vi "运维调试_五参数.vi"() -> ()   [LabVIEW 2016, in "斯坦道原位多参数.lvlib"]
uses:
  <vilib>/Utility/miscctls.llb/LVPointTypeDef.ctl
  <vilib>/Utility/config.llb/NI_LVConfig.lvlib
panel:
  in  "电导率单位":enum16{"mS/cm", "μS/cm"}(ring)
  in  "传感器类型":enum16{"STD自研", "纳清"}(ring)
  in  "校准":bool
  in  "获取传感器参数并保存触发":bool
  in  "传感器参数自动获取":bool=TRUE
  in  "标样测试组数":dbl=1.0 caption="标样测试组数:"
  in  "水样测试组数":dbl=1.0 caption="水样测试组数:"
  in  "转刷清洗时间":dbl=30.0 caption="转刷清洗时间:"
  in  "上电初始化时间":dbl=5.0 caption="上电初始化时间:"
  in  "水样稳定时间":dbl=5.0 caption="水样稳定时间:"
  out "串口号":string
  in  "水深写入":bool
  in  "水深读取":bool
  in  "水深校准":dbl caption="水深校准:"
  out "模块版本号":string
  in  "写入":bool
  in  "读取":bool
  in  "B":dbl caption="校准值B:"
  in  "K":dbl caption="校准值K:"
  in  "标样核查":bool
  in  "串口设置":bool
  in  "质控参数设置":bool
  in  "打开串口":bool
  in  "释放串口":bool
  out "多参数横条运行状态":T1(xcontrol)
  in  "数据区":i32(listbox)
  in  "停止测量(单探)":bool
  in  "启动测量(单探)":bool
  in  "控制命令区探头选择":u16(ring)=9 items=["氨氮"=3, "水温"=9, "pH值"=10, "溶解氧"=11, "电导率"=12, "浊度"=13, "叶绿素a"=14, "藻密度"=15, "蓝绿藻"=16, "氧化还原电位"=17, "溶解氧%"=18, "盐度"=19]
  in  "同步时间":bool
  in  "初始化(清洗)":bool
  in  "停止测量(全部)":bool
  in  "启动测量(全部)":bool
  in  "关键参数区读取":bool
  in  "关键参数区":i32(listbox)
  in  "传感器参数读取":bool
  in  "传感器区":i32(listbox)
  in  "返回":bool
  in  "设置":bool
  out "运行状态":string
  in  "停止":bool
  in  "水样测试":bool
  out "集成报警信息":string
  # "min"
  # "组"
  # "组"
  # "s"
  # "s"
  # "水深校准"
  # "控制命令区"
  # "探头校准"
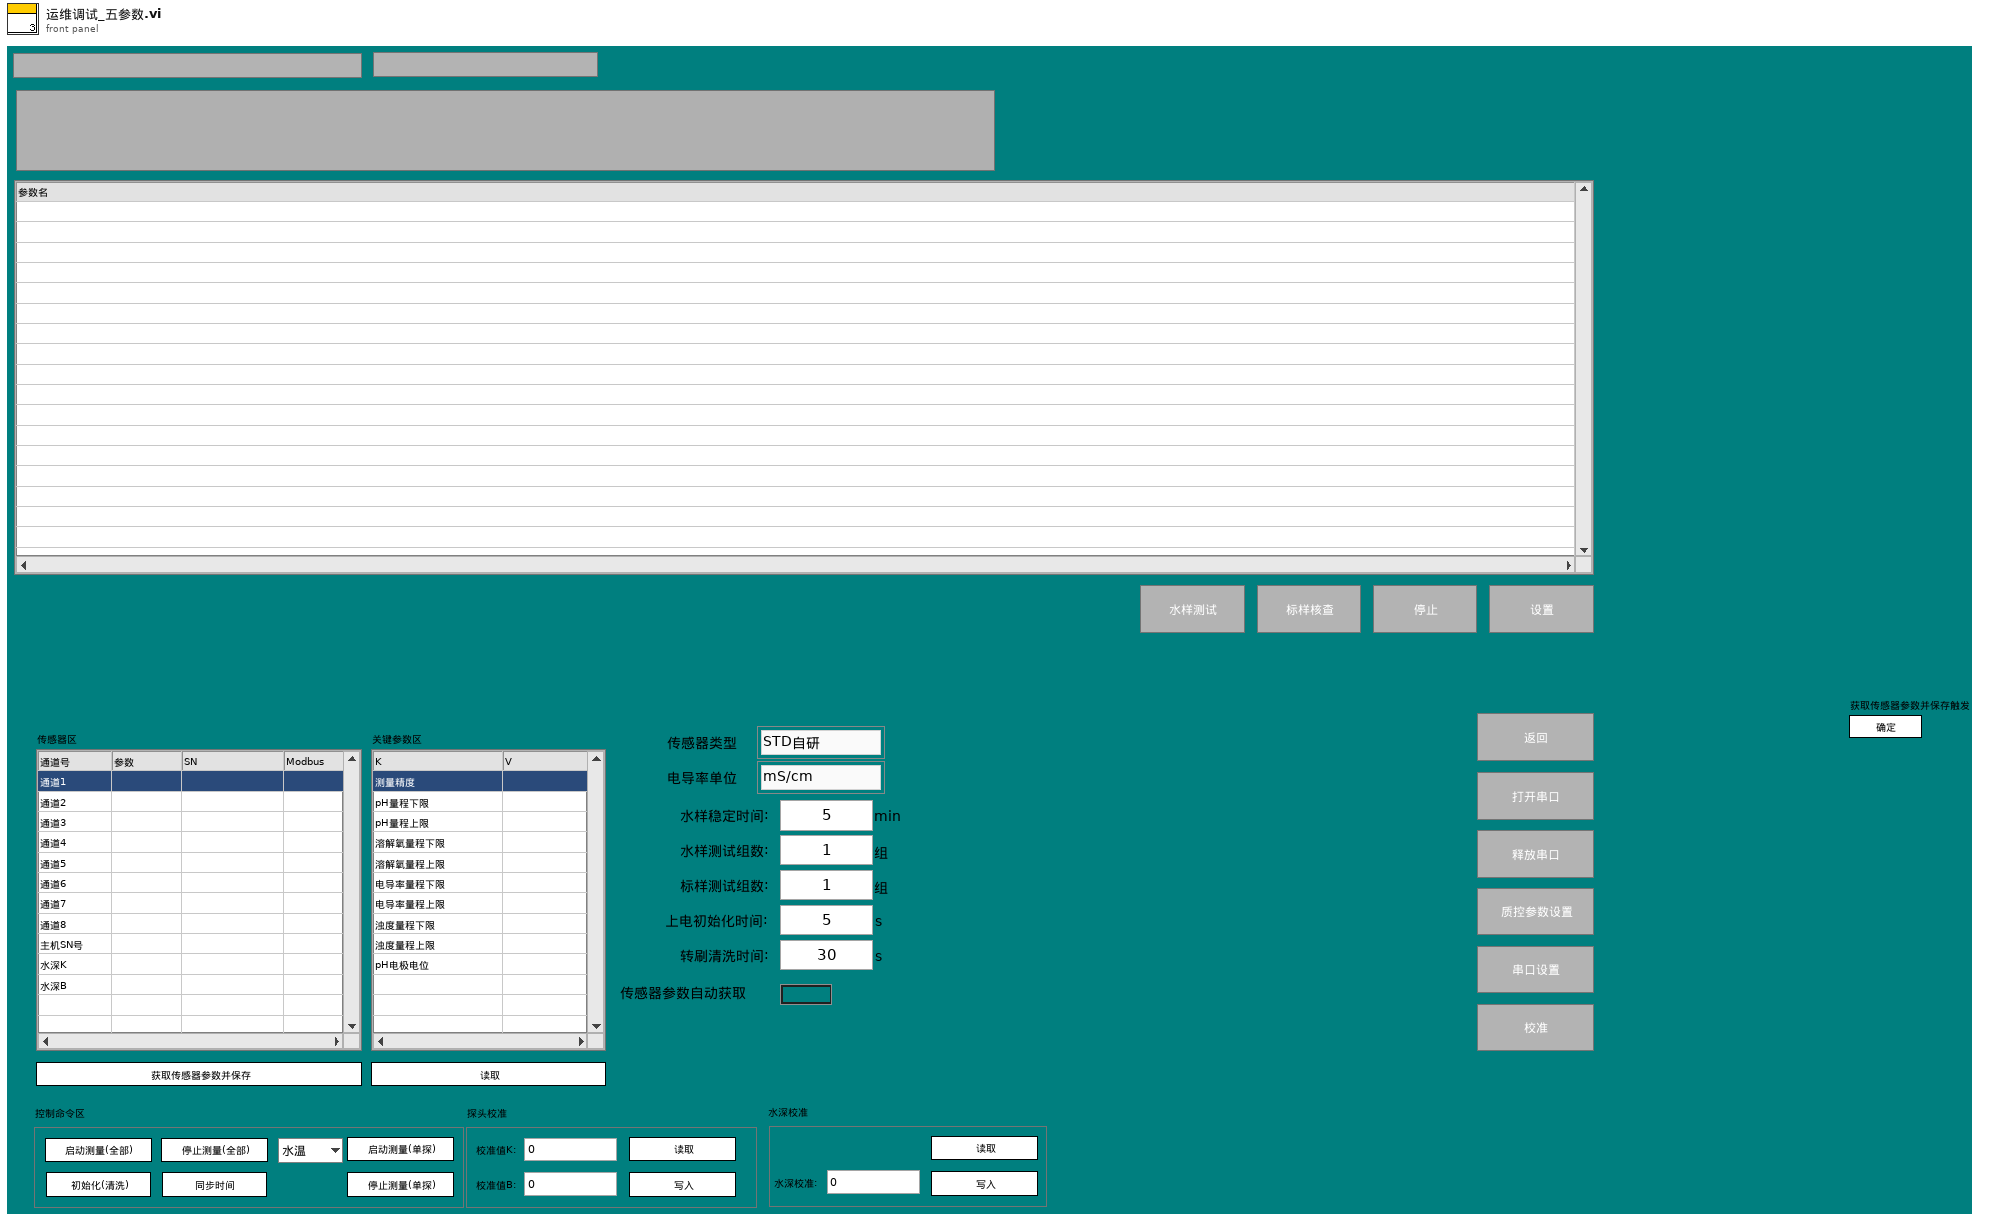
[diagram p1: front panel]
types:
  T1 = cluster{"系统时间":timestamp, "工作状态":u16, "测量模式":u16, "告警代码":enum16{"无告警", "缺试剂告警", "缺水样告警", "缺蒸馏水告警", "缺标液告警", "仪表漏液告警", "标定异常告警", "超量程告警", "加热异常", "低试剂预警", "超上限告警", "超下限告警", "仪表内部其他异常", "滴定异常告警", "电极异常告警", "量程切换告警", "参数设置告警", "PH电极电位异常", "电导率电极异常", "浊度光度异常", "溶解氧电极异常", "溶解氧光强异常", "温度异常告警", "PH异常告警", "溶解氧异常告警", "电导率异常告警", "浊度异常告警", "叶绿素异常告警", "藻密度异常告警", "蓝绿藻异常告警", "ORP异常告警", "氨氮异常告警", "清洁刷异常告警", "SD卡异常告警", "蓝牙异常告警", "Wifi异常告警", "流程异常告警"}, "故障代码":enum16{"无故障", "电机故障", "温度故障", "通讯故障", "滴定故障"}, "日志代码":u16, "软件版本":string}
  T2 = typedef "LVPointTypeDef.ctl" = cluster{"Horizontal":i16, "Vertical":i16}
  T3 = typedef "报警信息字段定义.ctl" = cluster{"时间":timestamp, "参数":string, "报警信息":string, "备注":string}
  T4 = enum16{"无告警", "缺试剂告警", "缺水样告警", "缺蒸馏水告警", "缺标液告警", "仪表漏液告警", "标定异常告警", "超量程告警", "加热异常", "低试剂预警", "超上限告警", "超下限告警", "仪表内部其他异常", "滴定异常告警", "电极异常告警", "量程切换告警", "参数设置告警", "PH电极电位异常", "电导率电极异常", "浊度光度异常", "溶解氧电极异常", "溶解氧光强异常", "温度异常告警", "PH异常告警", "溶解氧异常告警", "电导率异常告警", "浊度异常告警", "叶绿素异常告警", "藻密度异常告警", "蓝绿藻异常告警", "ORP异常告警", "氨氮异常告警", "清洁刷异常告警", "SD卡异常告警", "蓝牙异常告警", "Wifi异常告警", "流程异常告警"}
  T5 = cluster{"水温":dbl, "pH":dbl, "DO":dbl, "Cond":dbl, "Turb":dbl, "叶绿素":dbl, "藻密度":dbl, "蓝绿藻":dbl, "ORP":dbl, "NH3N":dbl}
  T6 = cluster{"因子编码":string, "单位":string, "标样参考值":sgl, "水样数据时间":timestamp, "水样实测值":sgl, "水样数据标识":string, "K":sgl, "B":sgl, "T":sgl, "H":sgl, "水深":sgl, "探头温度":sgl, "信号值":sgl}
  T7 = cluster{"Major":u16, "Minor":u16, "Fix":u16, "Build":u16}
  T8 = enum8{"Enabled", "Disabled", "Disabled and Grayed Out"}
  T9 = typedef "斯坦道原位多参数.lvlib/水样测试启动自定义输入参数.ctl" = cluster{"测量模式":string, "数据类型":string}
  T10 = typedef "斯坦道原位多参数.lvlib/标样核查启动自定义输入参数.ctl" = cluster{"测量模式":string, "数据类型":string, "输出参数":cluster{"水温":bool, "pH":bool, "DO":bool, "浊度":bool, "电导率":bool, "叶绿素a":bool, "蓝绿藻":bool, "藻密度":bool, "ORP":bool}}
  T11 = typedef "NI_LVConfig.lvlib/Config Data RefNum.ctl" = refnum<k1>
  T12 = cluster{"水温标准液标准浓度":dbl, "酸碱度标准液标准浓度":dbl, "溶解氧标准液标准浓度":dbl, "电导率标准液标准浓度":dbl, "浊度标准液标准浓度":dbl, "叶绿素a标准液标准浓度":dbl, "蓝绿藻标准液标准浓度":dbl, "ORP标准液标准浓度":dbl, "藻密度标准液标准浓度":dbl}
  T13 = cluster{"运行模式":enum16{"维护模式", "常规模式", "应急模式", "质控模式"}, "24H周期设置":bool[]}
  T14 = cluster{"水温":bool, "pH":bool, "DO":bool, "浊度":bool, "电导率":bool, "叶绿素a":bool, "蓝绿藻":bool, "藻密度":bool, "ORP":bool}
  T15 = enum32{"Bad", "Idle", "Run top level", "Running"}
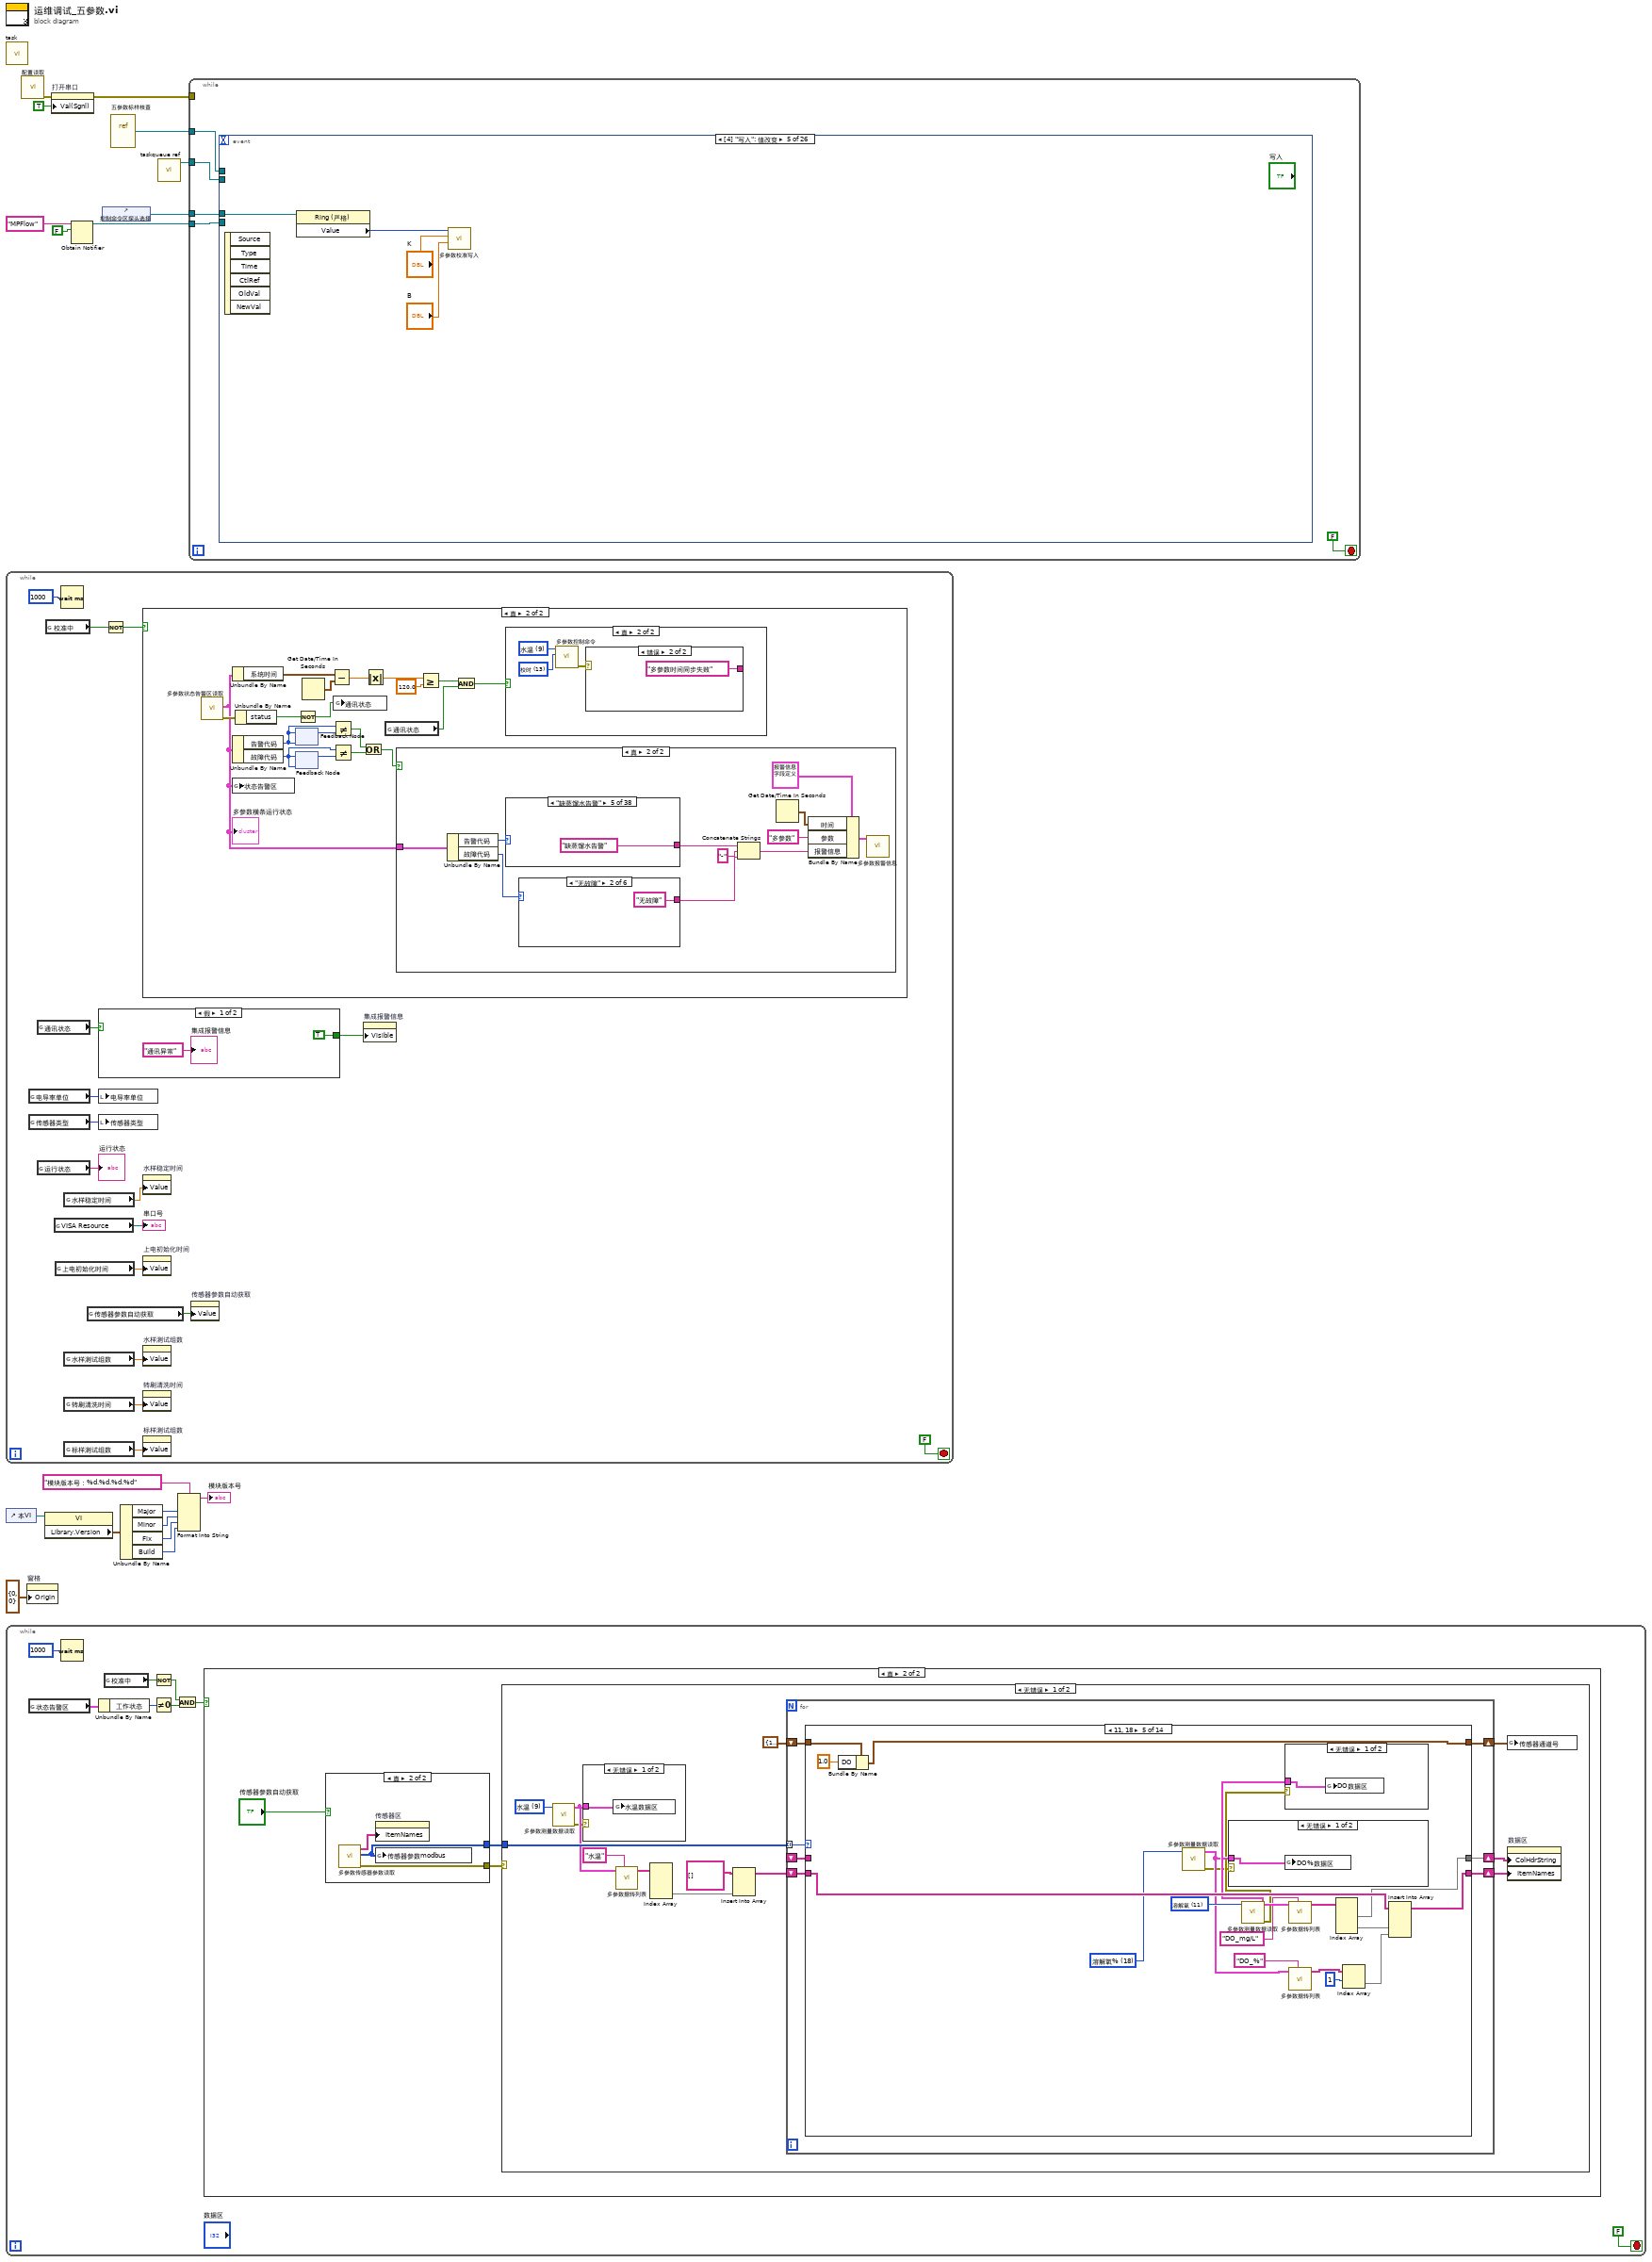
[diagram p0: block diagram]
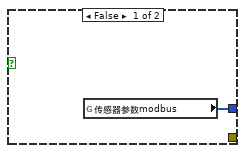
[diagram p3: hidden frame]
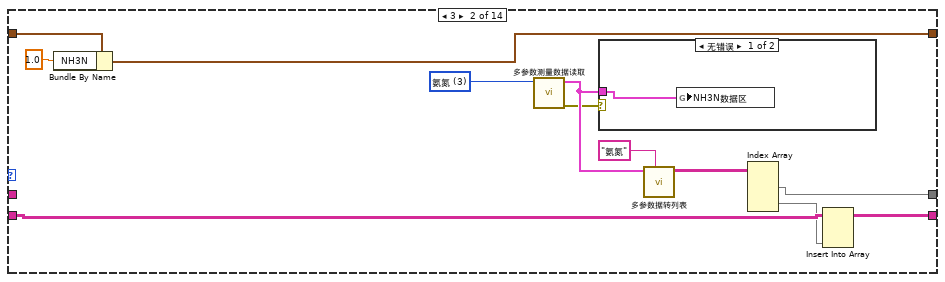
[diagram p6: hidden frame]
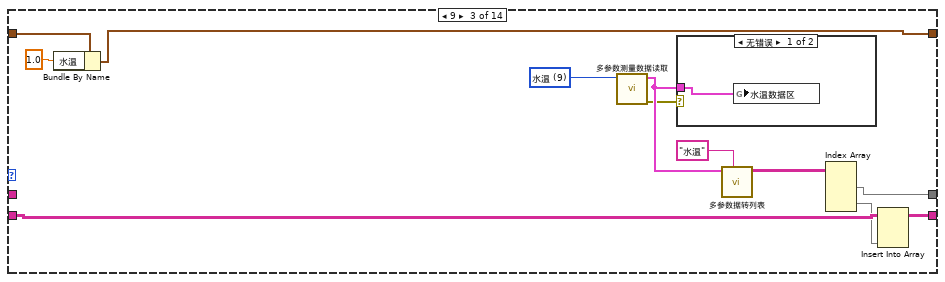
[diagram p8: hidden frame]
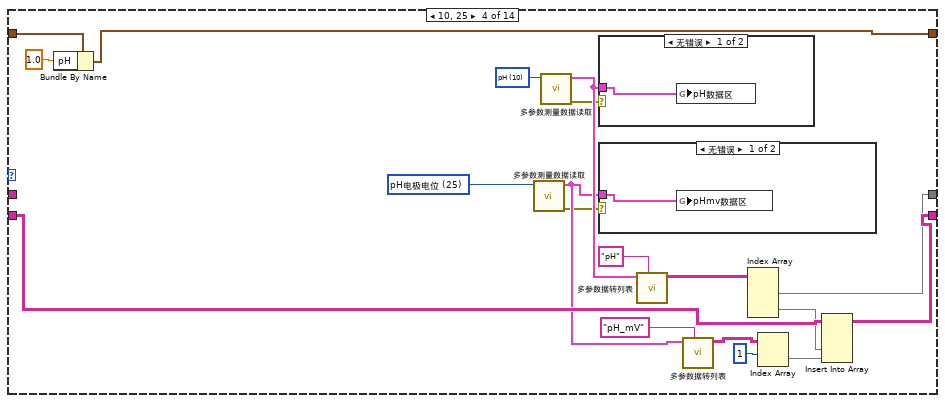
[diagram p10: hidden frame]
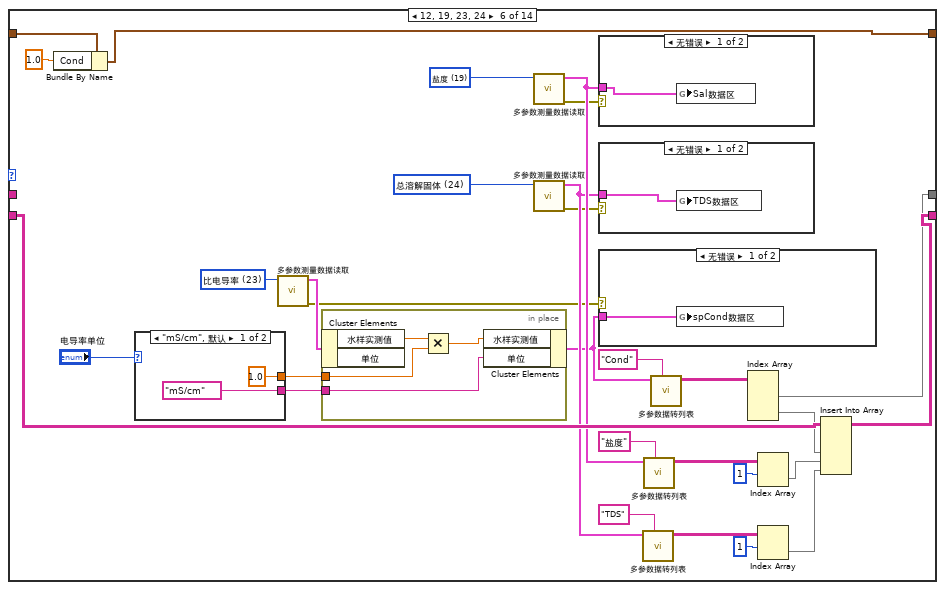
[diagram p15: hidden frame]
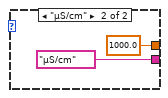
[diagram p16: hidden frame]
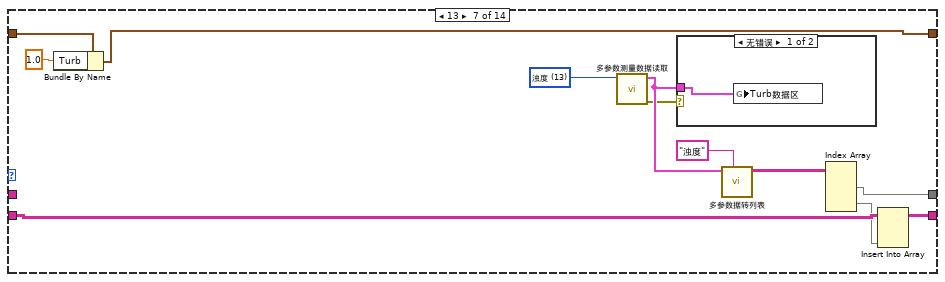
[diagram p20: hidden frame]
diagram:
  n1 = call "task.vi"() -> ()  [unwired: 12 in]
  n2 = while {
    stop <- FALSE stop-if-true
    n3 = global read "多参数断电保存全局变量.vi" "电导率单位"() -> (w21:enum16{"mS/cm", "μS/cm"})
    n4 = global read "多参数断电保存全局变量.vi" "传感器类型"() -> (w22:enum16{"STD自研", "纳清"})
    n5 = global read "多参数全局变量.vi" "通讯状态"() -> (w32:bool)
    n6 = global read "多参数全局变量.vi" "运行状态"() -> (→"运行状态":string)
    n7 = global read "多参数全局变量.vi" "校准中"() -> (w20:bool)
    n8 = global read "多参数断电保存全局变量.vi" "VISA Resource"() -> (→"串口号":refnum<visa-resource-name>)
    n9 = global read "多参数断电保存全局变量.vi" "上电初始化时间"() -> (w26:dbl)
    n10 = Wait (ms)(milliseconds to wait=u32 1000 ("等待时间（毫秒）")) -> ()  [unwired: 1 out]
    n11 = global read "多参数断电保存全局变量.vi" "水样稳定时间"() -> (w28:dbl)
    n12 = global read "多参数断电保存全局变量.vi" "水样测试组数"() -> (w27:dbl)
    n13 = global read "多参数断电保存全局变量.vi" "转刷清洗时间"() -> (w25:dbl)
    n14 = global read "多参数断电保存全局变量.vi" "标样测试组数"() -> (w24:dbl)
    n15 = global read "多参数断电保存全局变量.vi" "传感器参数自动获取"() -> (w23:bool)
    n16 = case shown="假" w32 {
      tunnel: [TRUE ("可见") _] -> w31
      frame False {
        "集成报警信息" <- "通讯异常" ("集成报警信息")
      }
      frame True {
      }
    }
    n17 = local write "电导率单位"(w21) -> ()
    n18 = local write "传感器类型"(w22) -> ()
    n19 = Not(x=w20) -> (.not. x?=w19:bool)
    n20 = case shown="真" w19 {
      frame False {
      }
      frame True {
        n21 = call "多参数状态告警区读取.vi"() -> ("error out"=w46:errorcluster, "状态告警块"=w43:T1)  [unwired: 9 in, 1 out]
        "多参数横条运行状态" <- w43
        n22 = Unbundle By Name(w43) -> ("系统时间"=w42:timestamp)
        n23 = Unbundle By Name(w43) -> ("告警代码"=w52:T4, "故障代码"=w50:enum16{"无故障", "电机故障", "温度故障", "通讯故障", "滴定故障"})
        n24 = global write "多参数全局变量.vi" "状态告警区"(w43) -> ()
        n25 = Unbundle By Name(w46) -> ("status"=w45:bool)
        n26 = feedback #1(w52) -> (w53:T4)
        n27 = feedback-in #1(w52) -> ()
        n28 = feedback #2(w50) -> (w51:enum16{"无故障", "电机故障", "温度故障", "通讯故障", "滴定故障"})
        n29 = feedback-in #2(w50) -> ()
        n30 = Not(x=w45) -> (.not. x?=w44:bool)
        n31 = Get Date/Time In Seconds() -> (seconds since 1Jan1904=w41:timestamp)
        n32 = Subtract(x=w42, y=w41) -> (x-y=w40:dbl)
        n33 = Not Equal?(x=w52, y=w53) -> (x != y?=w48:bool)
        n34 = Not Equal?(x=w50, y=w51) -> (x != y?=w49:bool)
        n35 = global write "多参数全局变量.vi" "通讯状态"(w44) -> ()
        n36 = Or(x=w48, y=w49) -> (x .or. y?=w47:bool)
        n37 = Absolute Value(x=w40) -> (abs(x)=w39:dbl)
        n38 = global read "多参数全局变量.vi" "通讯状态"() -> (w35:bool)
        n39 = case shown="真" w47 {
          tunnel: w43 -> [_ w69]
          frame False {
          }
          frame True {
            n40 = Unbundle By Name(w69) -> ("告警代码"=w68:T4, "故障代码"=w67:enum16{"无故障", "电机故障", "温度故障", "通讯故障", "滴定故障"})
            n41 = case shown="\"缺蒸馏水告警\"" w68 {
              selector: w68 -> [w80 _ _ _ _ _ _ _ _ _ _ _ _ _ _ _ _ _ _ _ _ _ _ _ _ _ _ _ _ _ _ _ _ _ _ _ _ _]
              tunnel: [w79 "无告警" "缺试剂告警" "缺水样告警" "缺蒸馏水告警" "缺标液告警" "仪表漏液告警" "标定异常告警" "超量程告警" "加热异常" "低试剂预警" "超上限告警" "超下限告警" "仪表内部其他异常" "滴定异常告警" "电极异常告警" "量程切换告警" "参数设置告警" "PH电极电位异常" "电导率电极异常" "浊度光度异常" "溶解氧电极异常" "溶解氧光强异常" "温度异常告警" "PH异常告警" "溶解氧异常告警" "电导率异常告警" "浊度异常告警" "叶绿素异常告警" "藻密度异常告警" "蓝绿藻异常告警" "ORP异常告警" "氨氮异常告警" "清洁刷异常告警" "SD卡异常告警" "蓝牙异常告警" "WiFi异常告警" "流程异常告警"] -> w66
              frame Default {
                n42 = Format Into String(format string="%d" ("格式字符串"), initial string="未知" ("工作状态"), w80) -> (resulting string=w79:string)  [unwired: 1 in, 1 out]
              }
              frame "无告警" {
              }
              frame "缺试剂告警" {
              }
              frame "缺水样告警" {
              }
              frame "缺蒸馏水告警" {
              }
              frame "缺标液告警" {
              }
              frame "仪表漏液告警" {
              }
              frame "标定异常告警" {
              }
              frame "超量程告警" {
              }
              frame "加热异常" {
              }
              frame "低试剂预警" {
              }
              frame "超上限告警" {
              }
              frame "超下限告警" {
              }
              frame "仪表内部其他异常" {
              }
              frame "滴定异常告警" {
              }
              frame "电极异常告警" {
              }
              frame "量程切换告警" {
              }
              frame "参数设置告警" {
              }
              frame "PH电极电位异常" {
              }
              frame "电导率电极异常" {
              }
              frame "浊度光度异常" {
              }
              frame "溶解氧电极异常" {
              }
              frame "溶解氧光强异常" {
              }
              frame "温度异常告警" {
              }
              frame "PH异常告警" {
              }
              frame "溶解氧异常告警" {
              }
              frame "电导率异常告警" {
              }
              frame "浊度异常告警" {
              }
              frame "叶绿素异常告警" {
              }
              frame "藻密度异常告警" {
              }
              frame "蓝绿藻异常告警" {
              }
              frame "ORP异常告警" {
              }
              frame "氨氮异常告警" {
              }
              frame "清洁刷异常告警" {
              }
              frame "SD卡异常告警" {
              }
              frame "蓝牙异常告警" {
              }
              frame "Wifi异常告警" {
              }
              frame "流程异常告警" {
              }
            }
            n43 = case shown="\"无故障\"" w67 {
              selector: w67 -> [w71 _ _ _ _ _]
              tunnel: [w70 "无故障" "电机故障" "温度故障" "通讯故障" "滴定故障"] -> w65
              frame Default {
                n44 = Format Into String(format string="%d" ("格式字符串"), initial string="未知" ("工作状态"), w71) -> (resulting string=w70:string)  [unwired: 1 in, 1 out]
              }
              frame "无故障" {
              }
              frame "电机故障" {
              }
              frame "温度故障" {
              }
              frame "通讯故障" {
              }
              frame "滴定故障" {
              }
            }
            n45 = Concatenate Strings(w66, "-" ("字符串"), w65) -> (w63:string)
            n46 = Get Date/Time In Seconds() -> (seconds since 1Jan1904=w62:timestamp)
            n47 = Bundle By Name(cluster=T3 {"时间"=timestamp(0 s since 1904-01-01), "参数"="", "报警信息"="", "备注"=""} ("data"), "时间"=w62, "参数"="多参数" ("设备"), "报警信息"=w63) -> (w59:T3)
            n48 = call "多参数报警信息.vi"("data"=w59) -> ()  [unwired: 10 in, 1 out]
          }
        }
        n49 = Greater Or Equal?(x=w39, y=120.0) -> (x >= y?=w38:bool)
        n50 = And(x=w38, y=w35) -> (x .and. y?=w36:bool)
        n51 = case shown="真" w36 {
          frame False {
          }
          frame True {
            w54 = u16 13 items=["启动测量（全部）"=1, "初始化（清洗）"=10, "停止测量（全部）"=11, "校时"=13, "启动测量（单个传感器）"=19, "停止测量（单个传感器）"=20] ("控制命令")
            w55 = u16 9 items=["氨氮"=3, "水温"=9, "pH值"=10, "溶解氧"=11, "电导率"=12, "浊度"=13, "叶绿素a"=14, "藻密度"=15, "蓝绿藻"=16, "氧化还原电位"=17, "溶解氧%"=18, "盐度"=19] ("站号")
            n52 = call "多参数控制命令.vi"("控制命令"=w54, "站号"=w55) -> ("error out"=w56:errorcluster)  [unwired: 9 in]
            n53 = case shown="错误" w56 {
              tunnel: ["多参数时间同步成功" ("消息") "多参数时间同步失败" ("消息")] -> _
              frame No Error {
              }
              frame Error {
              }
            }
          }
        }
      }
    }
    n54 = property on="水样稳定时间" class="DigNum (严格)"("Value"=w28) -> ()  [unwired: 2 in, 2 out]
    n55 = property on="上电初始化时间" class="DigNum (严格)"("Value"=w26) -> ()  [unwired: 2 in, 2 out]
    n56 = property on="水样测试组数" class="DigNum (严格)"("Value"=w27) -> ()  [unwired: 2 in, 2 out]
    n57 = property on="转刷清洗时间" class="DigNum (严格)"("Value"=w25) -> ()  [unwired: 2 in, 2 out]
    n58 = property on="标样测试组数" class="DigNum (严格)"("Value"=w24) -> ()  [unwired: 2 in, 2 out]
    n59 = property on="传感器参数自动获取" class="Bool (严格)"("Value"=w23) -> ()  [unwired: 2 in, 2 out]
    n60 = property on="集成报警信息" class="Str"("Visible"=w31) -> ()  [unwired: 2 in, 2 out]
  }
  n61 = control-ref of="本VI"() -> (w10:refnum<vi>)
  n62 = while {
    stop <- FALSE stop-if-true
    n63 = global read "多参数全局变量.vi" "状态告警区"() -> (w127:T1)
    n64 = Wait (ms)(milliseconds to wait=u32 1000 ("等待时间（毫秒）")) -> ()  [unwired: 1 out]
    n65 = Unbundle By Name(w127) -> ("工作状态"=w126:u16)
    n66 = global read "多参数全局变量.vi" "校准中"() -> (w124:bool)
    n67 = Not(x=w124) -> (.not. x?=w122:bool)
    n68 = Not Equal To 0?(x=w126) -> (x != 0?=w125:bool)
    n69 = And(x=w122, y=w125) -> (x .and. y?=w123:bool)
    n70 = case shown="真" w123 {
      frame False {
      }
      frame True {
        n71 = case shown="真" "传感器参数自动获取" {
          tunnel: [_ w136] -> w132
          tunnel: [w133 w134] -> w131
          frame False {
            n72 = global read "多参数断电保存全局变量.vi" "传感器参数modbus"() -> (w133:u16[])
          }
          frame True {
            n73 = call "多参数传感器参数读取.vi"() -> ("error out"=w136:errorcluster, "modbus"=w134:u16[], "添加的数组"=w135:string[][])  [unwired: 9 in]
            n74 = property on="传感器区" class="MCListbox (严格)"("ItemNames"=w135) -> ()  [unwired: 2 in, 2 out]
            n75 = global write "多参数断电保存全局变量.vi" "传感器参数modbus"(w134) -> ()
          }
        }
        n76 = case shown="无错误" w132 {
          tunnel: w131 -> [w149 _]
          frame No Error {
            w146 = u16 9 items=["氨氮"=3, "水温"=9, "pH"=10, "溶解氧"=11, "电导率"=12, "浊度"=13, "叶绿素a"=14, "藻密度"=15, "蓝绿藻"=16, "氧化还原电位"=17, "溶解氧%"=18, "盐度"=19, "水中油"=20, "高锰酸盐指数"=21, "化学需氧量"=22, "比电导率"=23, "总溶解固体"=24, "pH电极电位"=25] ("下拉列表")
            n77 = call "多参数测量数据读取.vi"("探头选择"=w146) -> ("error out"=w137:errorcluster, "测量数据块"=w141:T6)  [unwired: 8 in, 1 out]
            n78 = case shown="无错误" w137 {
              tunnel: w141 -> [w150 _]
              frame No Error {
                n79 = global write "多参数全局变量.vi" "水温数据区"(w150) -> ()
              }
              frame Error {
              }
            }
            n80 = call "多参数据转列表.vi"("参数名"="水温", "测量数据块"=w141) -> ("添加的数组"=w139:string[][])  [unwired: 9 in]
            n81 = Index Array(array=w139) -> (element #2=w138:string[])  [unwired: 4 in, 1 out]
            n82 = Insert Into Array(array=string[][] [] ("子数组"), new element=w138) -> (w144:string[][])  [unwired: 2 in]
            n83 = for {
              tunnel: w149 -> [w157] mode=indexing
              shift-right: [w155] -> w147
              shift-left: w144 -> [w156]
              shift-right: [w154] -> w148
              shift-left: _ -> [w153]
              shift-right: [w152] -> w142
              shift-left: T5 {"水温"=1.0, "pH"=0.0, "DO"=0.0, "Cond"=0.0, "Turb"=0.0, "叶绿素"=0.0, "藻密度"=0.0, "蓝绿藻"=0.0, "ORP"=0.0, "NH3N"=0.0} ("传感器通道号") -> [w151]
              n84 = case shown="11, 18" w157 {
                tunnel: w156 -> [w160 w171 w184 w204 w225 w257 w280 w293 w306 w319 w332 w342 w351 w360]
                tunnel: [w160 w170 w183 w203 w224 w256 w279 w292 w305 w318 w331 w341 w350 w359] -> w155
                tunnel: [w159 w163 w176 w196 w217 w248 w273 w285 w300 w312 w325 w336 w345 w354] -> w154
                tunnel: w153 -> [w159 _ _ _ _ _ _ _ _ _ _ _ _ _]
                tunnel: [w158 w167 w180 w199 w221 w251 w276 w289 w302 w315 w328 w340 w349 w358] -> w152
                tunnel: w151 -> [w158 w169 w182 w201 w223 w252 w277 w290 w303 w316 w329 w340 w349 w358]
                frame 0, Default {
                }
                frame 3 {
                  w172 = u16 3 items=["氨氮"=3, "水温"=9, "pH"=10, "溶解氧"=11, "电导率"=12, "浊度"=13, "叶绿素a"=14, "藻密度"=15, "蓝绿藻"=16, "氧化还原电位"=17, "溶解氧%"=18, "盐度"=19, "水中油"=20, "高锰酸盐指数"=21, "化学需氧量"=22, "比电导率"=23, "总溶解固体"=24, "pH电极电位"=25] ("下拉列表")
                  n85 = Bundle By Name(cluster=w169, "NH3N"=1.0) -> (w167:T5)
                  n86 = call "多参数测量数据读取.vi"("探头选择"=w172) -> ("error out"=w161:errorcluster, "测量数据块"=w166:T6)  [unwired: 8 in, 1 out]
                  n87 = case shown="无错误" w161 {
                    tunnel: w166 -> [w173 _]
                    frame No Error {
                      n88 = global write "多参数全局变量.vi" "NH3N数据区"(w173) -> ()
                    }
                    frame Error {
                    }
                  }
                  n89 = call "多参数据转列表.vi"("参数名"="氨氮", "测量数据块"=w166) -> ("添加的数组"=w165:string[][])  [unwired: 9 in]
                  n90 = Index Array(array=w165) -> (element #1=w163:string[], element #2=w162:string[])  [unwired: 4 in]
                  n91 = Insert Into Array(array=w171, new element=w162) -> (w170:string[][])  [unwired: 2 in]
                }
                frame 9 {
                  w185 = u16 9 items=["氨氮"=3, "水温"=9, "pH"=10, "溶解氧"=11, "电导率"=12, "浊度"=13, "叶绿素a"=14, "藻密度"=15, "蓝绿藻"=16, "氧化还原电位"=17, "溶解氧%"=18, "盐度"=19, "水中油"=20, "高锰酸盐指数"=21, "化学需氧量"=22, "比电导率"=23, "总溶解固体"=24, "pH电极电位"=25] ("下拉列表")
                  n92 = Bundle By Name(cluster=w182, "水温"=1.0) -> (w180:T5)
                  n93 = call "多参数测量数据读取.vi"("探头选择"=w185) -> ("error out"=w174:errorcluster, "测量数据块"=w179:T6)  [unwired: 8 in, 1 out]
                  n94 = case shown="无错误" w174 {
                    tunnel: w179 -> [w186 _]
                    frame No Error {
                      n95 = global write "多参数全局变量.vi" "水温数据区"(w186) -> ()
                    }
                    frame Error {
                    }
                  }
                  n96 = call "多参数据转列表.vi"("参数名"="水温", "测量数据块"=w179) -> ("添加的数组"=w178:string[][])  [unwired: 9 in]
                  n97 = Index Array(array=w178) -> (element #1=w176:string[], element #2=w175:string[])  [unwired: 4 in]
                  n98 = Insert Into Array(array=w184, new element=w175) -> (w183:string[][])  [unwired: 2 in]
                }
                frame 10, 25 {
                  w202 = u16 25 items=["氨氮"=3, "水温"=9, "pH"=10, "溶解氧"=11, "电导率"=12, "浊度"=13, "叶绿素a"=14, "藻密度"=15, "蓝绿藻"=16, "氧化还原电位"=17, "溶解氧%"=18, "盐度"=19, "水中油"=20, "高锰酸盐指数"=21, "化学需氧量"=22, "比电导率"=23, "总溶解固体"=24, "pH电极电位"=25] ("下拉列表")
                  w205 = u16 10 items=["氨氮"=3, "水温"=9, "pH"=10, "溶解氧"=11, "电导率"=12, "浊度"=13, "叶绿素a"=14, "藻密度"=15, "蓝绿藻"=16, "氧化还原电位"=17, "溶解氧%"=18, "盐度"=19, "水中油"=20, "高锰酸盐指数"=21, "化学需氧量"=22, "比电导率"=23, "总溶解固体"=24, "pH电极电位"=25] ("下拉列表")
                  n99 = Bundle By Name(cluster=w201, "pH"=1.0) -> (w199:T5)
                  n100 = call "多参数测量数据读取.vi"("探头选择"=w202) -> ("error out"=w187:errorcluster, "测量数据块"=w192:T6)  [unwired: 8 in, 1 out]
                  n101 = call "多参数测量数据读取.vi"("探头选择"=w205) -> ("error out"=w188:errorcluster, "测量数据块"=w198:T6)  [unwired: 8 in, 1 out]
                  n102 = case shown="无错误" w188 {
                    tunnel: w198 -> [w207 _]
                    frame No Error {
                      n103 = global write "多参数全局变量.vi" "pH数据区"(w207) -> ()
                    }
                    frame Error {
                    }
                  }
                  n104 = case shown="无错误" w187 {
                    tunnel: w192 -> [w206 _]
                    frame No Error {
                      n105 = global write "多参数全局变量.vi" "pHmv数据区"(w206) -> ()
                    }
                    frame Error {
                    }
                  }
                  n106 = call "多参数据转列表.vi"("参数名"="pH", "测量数据块"=w198) -> ("添加的数组"=w197:string[][])  [unwired: 9 in]
                  n107 = call "多参数据转列表.vi"("参数名"="pH_mV", "测量数据块"=w192) -> ("添加的数组"=w191:string[][])  [unwired: 9 in]
                  n108 = Index Array(array=w197) -> (element #1=w196:string[], element #2=w195:string[])  [unwired: 4 in]
                  n109 = Index Array(array=w191, index (row)=1 ("禁用的索引 (列)")) -> (element=w194:string[])  [unwired: 1 in]
                  n110 = Insert Into Array(array=w204, new element #1=w195, new element #2=w194) -> (w203:string[][])  [unwired: 2 in]
                }
                frame 11, 18 {
                  w215 = u16 18 items=["氨氮"=3, "水温"=9, "pH"=10, "溶解氧"=11, "电导率"=12, "浊度"=13, "叶绿素a"=14, "藻密度"=15, "蓝绿藻"=16, "氧化还原电位"=17, "溶解氧%"=18, "盐度"=19, "水中油"=20, "高锰酸盐指数"=21, "化学需氧量"=22, "比电导率"=23, "总溶解固体"=24, "pH电极电位"=25] ("下拉列表")
                  w226 = u16 11 items=["氨氮"=3, "水温"=9, "pH"=10, "溶解氧"=11, "电导率"=12, "浊度"=13, "叶绿素a"=14, "藻密度"=15, "蓝绿藻"=16, "氧化还原电位"=17, "溶解氧%"=18, "盐度"=19, "水中油"=20, "高锰酸盐指数"=21, "化学需氧量"=22, "比电导率"=23, "总溶解固体"=24, "pH电极电位"=25] ("下拉列表")
                  n111 = Bundle By Name(cluster=w223, "DO"=1.0) -> (w221:T5)
                  n112 = call "多参数测量数据读取.vi"("探头选择"=w215) -> ("error out"=w208:errorcluster, "测量数据块"=w214:T6)  [unwired: 8 in, 1 out]
                  n113 = case shown="无错误" w208 {
                    tunnel: w214 -> [w227 _]
                    frame No Error {
                      n114 = global write "多参数全局变量.vi" "DO%数据区"(w227) -> ()
                    }
                    frame Error {
                    }
                  }
                  n115 = call "多参数测量数据读取.vi"("探头选择"=w226) -> ("error out"=w209:errorcluster, "测量数据块"=w220:T6)  [unwired: 8 in, 1 out]
                  n116 = case shown="无错误" w209 {
                    tunnel: w220 -> [w228 _]
                    frame No Error {
                      n117 = global write "多参数全局变量.vi" "DO数据区"(w228) -> ()
                    }
                    frame Error {
                    }
                  }
                  n118 = call "多参数据转列表.vi"("参数名"="DO_mg/L", "测量数据块"=w220) -> ("添加的数组"=w218:string[][])  [unwired: 9 in]
                  n119 = call "多参数据转列表.vi"("参数名"="DO_%", "测量数据块"=w214) -> ("添加的数组"=w212:string[][])  [unwired: 9 in]
                  n120 = Index Array(array=w218) -> (element #1=w217:string[], element #2=w216:string[])  [unwired: 4 in]
                  n121 = Index Array(array=w212, index (row)=1 ("禁用的索引 (列)")) -> (element=w211:string[])  [unwired: 1 in]
                  n122 = Insert Into Array(array=w225, new element #1=w216, new element #2=w211) -> (w224:string[][])  [unwired: 2 in]
                }
                frame 12, 19, 23, 24 {
                  w254 = u16 24 items=["氨氮"=3, "水温"=9, "pH"=10, "溶解氧"=11, "电导率"=12, "浊度"=13, "叶绿素a"=14, "藻密度"=15, "蓝绿藻"=16, "氧化还原电位"=17, "溶解氧%"=18, "盐度"=19, "水中油"=20, "高锰酸盐指数"=21, "化学需氧量"=22, "比电导率"=23, "总溶解固体"=24, "pH电极电位"=25] ("下拉列表")
                  w255 = u16 19 items=["氨氮"=3, "水温"=9, "pH"=10, "溶解氧"=11, "电导率"=12, "浊度"=13, "叶绿素a"=14, "藻密度"=15, "蓝绿藻"=16, "氧化还原电位"=17, "溶解氧%"=18, "盐度"=19, "水中油"=20, "高锰酸盐指数"=21, "化学需氧量"=22, "比电导率"=23, "总溶解固体"=24, "pH电极电位"=25] ("下拉列表")
                  w258 = u16 23 items=["氨氮"=3, "水温"=9, "pH"=10, "溶解氧"=11, "电导率"=12, "浊度"=13, "叶绿素a"=14, "藻密度"=15, "蓝绿藻"=16, "氧化还原电位"=17, "溶解氧%"=18, "盐度"=19, "水中油"=20, "高锰酸盐指数"=21, "化学需氧量"=22, "比电导率"=23, "总溶解固体"=24, "pH电极电位"=25] ("下拉列表")
                  n123 = Bundle By Name(cluster=w252, "Cond"=1.0 ("DO")) -> (w251:T5)
                  n124 = case shown="\"mS/cm\", 默认" "电导率单位" {
                    tunnel: ["mS/cm" ("单位") "μS/cm" ("单位")] -> w230
                    tunnel: [sgl 1.0 ("y") sgl 1000.0 ("y")] -> w229
                    frame "mS/cm", Default {
                    }
                    frame "μS/cm" {
                    }
                  }
                  n125 = call "多参数测量数据读取.vi"("探头选择"=w258) -> ("error out"=w234:errorcluster, "测量数据块"=w240:T6)  [unwired: 8 in, 1 out]
                  n126 = in-place {
                    in-place-border: w230 -> [w267]
                    in-place-border: w229 -> [w266]
                    n127 = in-place-cluster #3(w240) -> ("水样实测值"=w269:sgl)  [unwired: 1 out]
                    n128 = Multiply(x=w269, y=w266) -> (x*y=w268:sgl)
                    n129 = in-place-cluster #3("水样实测值"=w268, "单位"=w267) -> (w239:T6)
                  }
                  n130 = call "多参数测量数据读取.vi"("探头选择"=w255) -> ("error out"=w233:errorcluster, "测量数据块"=w245:T6)  [unwired: 8 in, 1 out]
                  n131 = call "多参数测量数据读取.vi"("探头选择"=w254) -> ("error out"=w232:errorcluster, "测量数据块"=w242:T6)  [unwired: 8 in, 1 out]
                  n132 = case shown="无错误" w233 {
                    tunnel: w245 -> [w264 _]
                    frame No Error {
                      n133 = global write "多参数全局变量.vi" "Sal数据区"(w264) -> ()
                    }
                    frame Error {
                    }
                  }
                  n134 = case shown="无错误" w232 {
                    tunnel: w242 -> [w263 _]
                    frame No Error {
                      n135 = global write "多参数全局变量.vi" "TDS数据区"(w263) -> ()
                    }
                    frame Error {
                    }
                  }
                  n136 = case shown="无错误" w234 {
                    tunnel: w239 -> [w265 _]
                    frame No Error {
                      n137 = global write "多参数全局变量.vi" "spCond数据区"(w265) -> ()
                    }
                    frame Error {
                    }
                  }
                  n138 = call "多参数据转列表.vi"("参数名"="TDS", "测量数据块"=w242) -> ("添加的数组"=w241:string[][])  [unwired: 9 in]
                  n139 = call "多参数据转列表.vi"("参数名"="盐度", "测量数据块"=w245) -> ("添加的数组"=w244:string[][])  [unwired: 9 in]
                  n140 = call "多参数据转列表.vi"("参数名"="Cond", "测量数据块"=w239) -> ("添加的数组"=w249:string[][])  [unwired: 9 in]
                  n141 = Index Array(array=w249) -> (element #1=w248:string[], element #2=w247:string[])  [unwired: 4 in]
                  n142 = Index Array(array=w244, index (row)=1 ("禁用的索引 (列)")) -> (element=w236:string[])  [unwired: 1 in]
                  n143 = Index Array(array=w241, index (row)=1 ("禁用的索引 (列)")) -> (element=w235:string[])  [unwired: 1 in]
                  n144 = Insert Into Array(array=w257, new element #1=w247, new element #2=w236, new element #3=w235) -> (w256:string[][])  [unwired: 2 in]
                }
                frame 13 {
                  w281 = u16 13 items=["氨氮"=3, "水温"=9, "pH"=10, "溶解氧"=11, "电导率"=12, "浊度"=13, "叶绿素a"=14, "藻密度"=15, "蓝绿藻"=16, "氧化还原电位"=17, "溶解氧%"=18, "盐度"=19, "水中油"=20, "高锰酸盐指数"=21, "化学需氧量"=22, "比电导率"=23, "总溶解固体"=24, "pH电极电位"=25] ("下拉列表")
                  n145 = Bundle By Name(cluster=w277, "Turb"=1.0 ("DO")) -> (w276:T5)
                  n146 = call "多参数测量数据读取.vi"("探头选择"=w281) -> ("error out"=w270:errorcluster, "测量数据块"=w271:T6)  [unwired: 8 in, 1 out]
                  n147 = case shown="无错误" w270 {
                    tunnel: w271 -> [w282 _]
                    frame No Error {
                      n148 = global write "多参数全局变量.vi" "Turb数据区"(w282) -> ()
                    }
                    frame Error {
                    }
                  }
                  n149 = call "多参数据转列表.vi"("参数名"="浊度", "测量数据块"=w271) -> ("添加的数组"=w274:string[][])  [unwired: 9 in]
                  n150 = Index Array(array=w274) -> (element #1=w273:string[], element #2=w272:string[])  [unwired: 4 in]
                  n151 = Insert Into Array(array=w280, new element=w272) -> (w279:string[][])  [unwired: 2 in]
                }
                frame 14 {
                  w294 = u16 14 items=["氨氮"=3, "水温"=9, "pH"=10, "溶解氧"=11, "电导率"=12, "浊度"=13, "叶绿素a"=14, "藻密度"=15, "蓝绿藻"=16, "氧化还原电位"=17, "溶解氧%"=18, "盐度"=19, "水中油"=20, "高锰酸盐指数"=21, "化学需氧量"=22, "比电导率"=23, "总溶解固体"=24, "pH电极电位"=25] ("下拉列表")
                  n152 = Bundle By Name(cluster=w290, "叶绿素"=1.0 ("DO")) -> (w289:T5)
                  n153 = call "多参数测量数据读取.vi"("探头选择"=w294) -> ("error out"=w283:errorcluster, "测量数据块"=w288:T6)  [unwired: 8 in, 1 out]
                  n154 = case shown="无错误" w283 {
                    tunnel: w288 -> [w295 _]
                    frame No Error {
                      n155 = global write "多参数全局变量.vi" "叶绿素数据区"(w295) -> ()
                    }
                    frame Error {
                    }
                  }
                  n156 = call "多参数据转列表.vi"("参数名"="叶绿素a", "测量数据块"=w288) -> ("添加的数组"=w286:string[][])  [unwired: 9 in]
                  n157 = Index Array(array=w286) -> (element #1=w285:string[], element #2=w284:string[])  [unwired: 4 in]
                  n158 = Insert Into Array(array=w293, new element=w284) -> (w292:string[][])  [unwired: 2 in]
                }
                frame 15 {
                  w307 = u16 15 items=["氨氮"=3, "水温"=9, "pH"=10, "溶解氧"=11, "电导率"=12, "浊度"=13, "叶绿素a"=14, "藻密度"=15, "蓝绿藻"=16, "氧化还原电位"=17, "溶解氧%"=18, "盐度"=19, "水中油"=20, "高锰酸盐指数"=21, "化学需氧量"=22, "比电导率"=23, "总溶解固体"=24, "pH电极电位"=25] ("下拉列表")
                  n159 = Bundle By Name(cluster=w303, "藻密度"=1.0 ("DO")) -> (w302:T5)
                  n160 = call "多参数测量数据读取.vi"("探头选择"=w307) -> ("error out"=w296:errorcluster, "测量数据块"=w299:T6)  [unwired: 8 in, 1 out]
                  n161 = case shown="无错误" w296 {
                    tunnel: w299 -> [w308 _]
                    frame No Error {
                      n162 = global write "多参数全局变量.vi" "藻密度数据区"(w308) -> ()
                    }
                    frame Error {
                    }
                  }
                  n163 = call "多参数据转列表.vi"("参数名"="藻密度", "测量数据块"=w299) -> ("添加的数组"=w301:string[][])  [unwired: 9 in]
                  n164 = Index Array(array=w301) -> (element #1=w300:string[], element #2=w298:string[])  [unwired: 4 in]
                  n165 = Insert Into Array(array=w306, new element=w298) -> (w305:string[][])  [unwired: 2 in]
                }
                frame 16 {
                  w320 = u16 16 items=["氨氮"=3, "水温"=9, "pH"=10, "溶解氧"=11, "电导率"=12, "浊度"=13, "叶绿素a"=14, "藻密度"=15, "蓝绿藻"=16, "氧化还原电位"=17, "溶解氧%"=18, "盐度"=19, "水中油"=20, "高锰酸盐指数"=21, "化学需氧量"=22, "比电导率"=23, "总溶解固体"=24, "pH电极电位"=25] ("下拉列表")
                  n166 = Bundle By Name(cluster=w316, "蓝绿藻"=1.0 ("DO")) -> (w315:T5)
                  n167 = call "多参数测量数据读取.vi"("探头选择"=w320) -> ("error out"=w309:errorcluster, "测量数据块"=w314:T6)  [unwired: 8 in, 1 out]
                  n168 = case shown="无错误" w309 {
                    tunnel: w314 -> [w321 _]
                    frame No Error {
                      n169 = global write "多参数全局变量.vi" "蓝绿藻数据区"(w321) -> ()
                    }
                    frame Error {
                    }
                  }
                  n170 = call "多参数据转列表.vi"("参数名"="蓝绿藻", "测量数据块"=w314) -> ("添加的数组"=w313:string[][])  [unwired: 9 in]
                  n171 = Index Array(array=w313) -> (element #1=w312:string[], element #2=w311:string[])  [unwired: 4 in]
                  n172 = Insert Into Array(array=w319, new element=w311) -> (w318:string[][])  [unwired: 2 in]
                }
                frame 17 {
                  w333 = u16 17 items=["氨氮"=3, "水温"=9, "pH"=10, "溶解氧"=11, "电导率"=12, "浊度"=13, "叶绿素a"=14, "藻密度"=15, "蓝绿藻"=16, "氧化还原电位"=17, "溶解氧%"=18, "盐度"=19, "水中油"=20, "高锰酸盐指数"=21, "化学需氧量"=22, "比电导率"=23, "总溶解固体"=24, "pH电极电位"=25] ("下拉列表")
                  n173 = Bundle By Name(cluster=w329, "ORP"=1.0 ("DO")) -> (w328:T5)
                  n174 = call "多参数测量数据读取.vi"("探头选择"=w333) -> ("error out"=w322:errorcluster, "测量数据块"=w327:T6)  [unwired: 8 in, 1 out]
                  n175 = case shown="无错误" w322 {
                    tunnel: w327 -> [w334 _]
                    frame No Error {
                      n176 = global write "多参数全局变量.vi" "ORP数据区"(w334) -> ()
                    }
                    frame Error {
                    }
                  }
                  n177 = call "多参数据转列表.vi"("参数名"="ORP", "测量数据块"=w327) -> ("添加的数组"=w326:string[][])  [unwired: 9 in]
                  n178 = Index Array(array=w326) -> (element #1=w325:string[], element #2=w323:string[])  [unwired: 4 in]
                  n179 = Insert Into Array(array=w332, new element=w323) -> (w331:string[][])  [unwired: 2 in]
                }
                frame 20 {
                  w343 = u16 20 items=["氨氮"=3, "水温"=9, "pH"=10, "溶解氧"=11, "电导率"=12, "浊度"=13, "叶绿素a"=14, "藻密度"=15, "蓝绿藻"=16, "氧化还原电位"=17, "溶解氧%"=18, "盐度"=19, "水中油"=20, "高锰酸盐指数"=21, "化学需氧量"=22, "比电导率"=23, "总溶解固体"=24, "pH电极电位"=25] ("下拉列表")
                  n180 = call "多参数测量数据读取.vi"("探头选择"=w343) -> ("测量数据块"=w339:T6)  [unwired: 8 in, 2 out]
                  n181 = call "多参数据转列表.vi"("参数名"="水中油", "测量数据块"=w339) -> ("添加的数组"=w337:string[][])  [unwired: 9 in]
                  n182 = Index Array(array=w337) -> (element #1=w336:string[], element #2=w335:string[])  [unwired: 4 in]
                  n183 = Insert Into Array(array=w342, new element=w335) -> (w341:string[][])  [unwired: 2 in]
                }
                frame 21 {
                  w352 = u16 21 items=["氨氮"=3, "水温"=9, "pH"=10, "溶解氧"=11, "电导率"=12, "浊度"=13, "叶绿素a"=14, "藻密度"=15, "蓝绿藻"=16, "氧化还原电位"=17, "溶解氧%"=18, "盐度"=19, "水中油"=20, "高锰酸盐指数"=21, "化学需氧量"=22, "比电导率"=23, "总溶解固体"=24, "pH电极电位"=25] ("下拉列表")
                  n184 = call "多参数测量数据读取.vi"("探头选择"=w352) -> ("测量数据块"=w348:T6)  [unwired: 8 in, 2 out]
                  n185 = call "多参数据转列表.vi"("参数名"="高锰酸盐指数", "测量数据块"=w348) -> ("添加的数组"=w347:string[][])  [unwired: 9 in]
                  n186 = Index Array(array=w347) -> (element #1=w345:string[], element #2=w344:string[])  [unwired: 4 in]
                  n187 = Insert Into Array(array=w351, new element=w344) -> (w350:string[][])  [unwired: 2 in]
                }
                frame 22 {
                  w361 = u16 22 items=["氨氮"=3, "水温"=9, "pH"=10, "溶解氧"=11, "电导率"=12, "浊度"=13, "叶绿素a"=14, "藻密度"=15, "蓝绿藻"=16, "氧化还原电位"=17, "溶解氧%"=18, "盐度"=19, "水中油"=20, "高锰酸盐指数"=21, "化学需氧量"=22, "比电导率"=23, "总溶解固体"=24, "pH电极电位"=25] ("下拉列表")
                  n188 = call "多参数测量数据读取.vi"("探头选择"=w361) -> ("测量数据块"=w357:T6)  [unwired: 8 in, 2 out]
                  n189 = call "多参数据转列表.vi"("参数名"="化学需氧量", "测量数据块"=w357) -> ("添加的数组"=w356:string[][])  [unwired: 9 in]
                  n190 = Index Array(array=w356) -> (element #1=w354:string[], element #2=w353:string[])  [unwired: 4 in]
                  n191 = Insert Into Array(array=w360, new element=w353) -> (w359:string[][])  [unwired: 2 in]
                }
              }
            }
            n192 = global write "多参数全局变量.vi" "传感器通道号"(w142) -> ()
            n193 = property on="数据区" class="MCListbox (严格)"("ColHdrString"=w148, "ItemNames"=w147) -> ()  [unwired: 2 in, 2 out]
          }
          frame Error {
          }
        }
      }
    }
  }
  n194 = call "配置读取.vi"() -> ("error out"=w1:errorcluster)  [unwired: 11 in]
  n195 = property on="窗格" class="Pane"("Origin"=T2 {"Horizontal"=0, "Vertical"=0} ("原点")) -> ()  [unwired: 2 in, 2 out]
  n196 = property class="VI"(reference=w10) -> ("Library.Version"=w9:T7)  [unwired: 1 in, 2 out]
  n197 = property on="打开串口" class="Bool (严格)"(error in=w1, "Val(Sgnl)"=TRUE ("值(信号)")) -> (error out=w12:errorcluster)  [unwired: 1 in, 1 out]
  n198 = Obtain Notifier(name (unnamed)="MPFlow" ("名称（未命名）"), notification data type=FALSE) -> (notifier out=w15:refnum<notifier>)  [unwired: 2 in, 2 out]
  n199 = control-ref of="控制命令区探头选择"() -> (w14:refnum<vi>)
  n200 = vi-ref "五参数标样核查.vi"() -> (w11:refnum<vi>)
  n201 = Unbundle By Name(w9) -> ("Major"=w7:u16, "Minor"=w6:u16, "Fix"=w5:u16, "Build"=w4:u16)
  n202 = call "taskqueue ref.vi"() -> ("队列输出"=w2:refnum<queue>)  [unwired: 10 in, 1 out]
  n203 = Format Into String(format string="模块版本号：%d.%d.%d.%d" ("格式字符串"), w7, w6, w5, w4) -> (resulting string=→"模块版本号":string)  [unwired: 2 in, 1 out]
  n204 = while {
    tunnel: w15 -> [w365]
    tunnel: w14 -> [w364]
    tunnel: w12 -> [_]
    tunnel: w11 -> [w363]
    tunnel: w2 -> [w362]
    stop <- FALSE stop-if-true
    n205 = event shown="[4] \"写入\": 值改变" {
      selector: _ -> [_ _ _ _ _ _ _ _ _ _ _ _ _ _ _ _ _ _ _ _ _ _ _ _ _ _]
      dyn-events: _ -> [_ _ _ _ _ _ _ _ _ _ _ _ _ _ _ _ _ _ _ _ _ _ _ _ _ _]
      timeout: _ -> [_ _ _ _ _ _ _ _ _ _ _ _ _ _ _ _ _ _ _ _ _ _ _ _ _ _]
      tunnel: w365 -> [_ _ _ _ _ _ _ _ _ _ _ _ _ _ _ w484 _ _ _ _ _ _ _ _ _ _]
      tunnel: w364 -> [_ _ _ w375 w379 _ _ _ _ _ _ _ _ _ _ _ _ _ _ _ _ _ _ _ w527 w534]
      tunnel: w363 -> [_ _ _ _ _ _ _ _ _ _ _ _ _ _ w460 _ _ _ _ _ _ _ _ _ _ _]
      tunnel: w362 -> [_ _ _ _ _ _ _ _ _ _ _ _ _ w456 _ _ _ _ _ _ _ _ _ _ _ _]
      event Timeout {
        n206 = event-data() -> ()  [unwired: 1 in, 3 out]
      }
      event "校准": Value Change {
        n207 = event-data() -> ()  [unwired: 1 in, 6 out]
        n208 = global read "多参数断电保存全局变量.vi" "传感器类型"() -> (w367:enum16{"STD自研", "纳清"})
        n209 = case shown="\"STD自研\", 默认" w367 {
          frame "STD自研", Default {
            n210 = call "STD校准画面.vi"() -> ()  [unwired: 12 in]
          }
          frame "纳清" {
            n211 = call "校准画面.vi"() -> ()  [unwired: 12 in]
          }
        }
      }
      event "K", "B", "水深校准", "水样稳定时间", "上电初始化时间", "转刷清洗时间", "水样测试组数", "标样测试组数": Mouse Down {
        n212 = event-data() -> ("CtlRef"=w371:refnum<vi>)  [unwired: 1 in, 7 out]
        n213 = property class="DigNum (严格)"(reference=w371) -> (reference out=w369:refnum<vi>, "Value"=w370:dbl)  [unwired: 1 in, 1 out]
        n214 = call "数字键盘.vi"("OldNumber"=w370) -> ("NewNumber"=w368:dbl)
        n215 = property class="DigNum (严格)"(reference=w369, "Val(Sgnl)"=w368) -> ()  [unwired: 1 in, 2 out]
      }
      event "读取": Value Change {
        n216 = event-data() -> ()  [unwired: 1 in, 6 out]
        n217 = property class="Ring (严格)"(reference=w375) -> ("Value"=w374:u16)  [unwired: 1 in, 2 out]
        n218 = call "多参校准读取.vi"("站号"=w374) -> ("B"=w372:dbl, "K"=w373:dbl)  [unwired: 8 in, 1 out]
        n219 = local write "K"(w373) -> ()
        n220 = local write "B"(w372) -> ()
      }
      event "写入": Value Change {
        n221 = event-data() -> ()  [unwired: 1 in, 6 out]
        n222 = property class="Ring (严格)"(reference=w379) -> ("Value"=w378:u16)  [unwired: 1 in, 2 out]
        n223 = call "多参数校准写入.vi"("B"="B", "K"="K", "站号"=w378) -> ()  [unwired: 8 in, 1 out]
      }
      event "水深读取": Value Change {
        w381 = u16 9 items=["氨氮"=3, "水温"=9, "pH值"=10, "溶解氧"=11, "电导率"=12, "浊度"=13, "叶绿素a"=14, "藻密度"=15, "蓝绿藻"=16, "氧化还原电位"=17, "溶解氧%"=18, "盐度"=19] ("站号")
        n224 = event-data() -> ()  [unwired: 1 in, 6 out]
        n225 = call "多参水深校准读取.vi"("站号"=w381) -> ("B"=w380:dbl)  [unwired: 8 in, 2 out]
        n226 = local write "水深校准"(w380) -> ()
      }
      event "水深写入": Value Change {
        w383 = u16 9 items=["氨氮"=3, "水温"=9, "pH值"=10, "溶解氧"=11, "电导率"=12, "浊度"=13, "叶绿素a"=14, "藻密度"=15, "蓝绿藻"=16, "氧化还原电位"=17, "溶解氧%"=18, "盐度"=19] ("站号")
        n227 = event-data() -> ()  [unwired: 1 in, 6 out]
        n228 = call "多参数水深校准写入.vi"("K"="水深校准", "站号"=w383) -> ()  [unwired: 9 in, 1 out]
      }
      event "串口设置": Value Change {
        n229 = event-data() -> ()  [unwired: 1 in, 6 out]
        n230 = global read "多参数断电保存全局变量.vi" "VISA Resource"() -> (w388:refnum<visa-resource-name>)
        n231 = global read "多参数断电保存全局变量.vi" "波特率"() -> (w386:u32)
        n232 = call "串口配置.vi"("波特率"=w386, "VISA资源名称"=w388) -> ("确认 2"=w384:bool, "波特率 2"=w385:u32, "VISA资源名称 2"=w387:refnum<visa-resource-name>)  [unwired: 7 in]
        n233 = case shown="真" w384 {
          tunnel: w387 -> [_ w390]
          tunnel: w385 -> [_ w389]
          frame False {
          }
          frame True {
            n234 = flat-sequence {
              tunnel: w390 -> [w392]
              tunnel: w389 -> [w391]
              frame #0 {
                n235 = global write "多参数断电保存全局变量.vi" "VISA Resource"(w392) -> ()
                n236 = global write "多参数断电保存全局变量.vi" "波特率"(w391) -> ()
              }
              frame #1 {
                n237 = call "多参数通讯.vi"("STEP"=enum16{"open", "read", "write", "close"}."open") -> ("error out"=w394:errorcluster)  [unwired: 8 in, 2 out]
                n238 = case shown="错误" w394 {
                  frame No Error {
                  }
                  frame Error {
                    n239 = One Button Dialog(message="多参数串口打开失败" ("消息")) -> ()  [unwired: 1 in, 1 out]
                  }
                }
              }
              frame #2 {
                n240 = call "配置保存.vi"() -> ()  [unwired: 11 in, 1 out]
              }
            }
          }
        }
      }
      event "水样稳定时间", "上电初始化时间", "转刷清洗时间", "水样测试组数", "标样测试组数", "传感器类型", "电导率单位": Value Change {
        n241 = event-data() -> ()  [unwired: 1 in, 6 out]
        n242 = flat-sequence {
          frame #0 {
            n243 = local read "电导率单位"() -> (w396:enum16{"mS/cm", "μS/cm"})
            n244 = global write "多参数断电保存全局变量.vi" "电导率单位"(w396) -> ()
            n245 = global write "多参数断电保存全局变量.vi" "水样稳定时间"("水样稳定时间") -> ()
            n246 = global write "多参数断电保存全局变量.vi" "水样测试组数"("水样测试组数") -> ()
            n247 = global write "多参数断电保存全局变量.vi" "上电初始化时间"("上电初始化时间") -> ()
            n248 = global write "多参数断电保存全局变量.vi" "传感器类型"("传感器类型") -> ()
            n249 = global write "多参数断电保存全局变量.vi" "转刷清洗时间"("转刷清洗时间") -> ()
            n250 = global write "多参数断电保存全局变量.vi" "标样测试组数"("标样测试组数") -> ()
          }
          frame #1 {
            n251 = call "配置保存.vi"() -> ()  [unwired: 11 in, 1 out]
          }
        }
      }
      event "传感器参数自动获取": Value Change {
        n252 = event-data() -> ("NewVal"=w403:bool)  [unwired: 1 in, 5 out]
        n253 = case shown="假" w403 {
          frame False {
            n254 = property on="获取传感器参数并保存触发" class="Bool (严格)"("Val(Sgnl)"=FALSE ("获取传感器参数并保存触发")) -> ()  [unwired: 2 in, 2 out]
          }
          frame True {
          }
        }
        n255 = flat-sequence {
          tunnel: w403 -> [w405]
          frame #0 {
            n256 = global write "多参数断电保存全局变量.vi" "传感器参数自动获取"(w405) -> ()
          }
          frame #1 {
            n257 = call <vilib>:"Application Directory.vi"() -> ("Application Directory"=w419:path)
            n258 = Build Path(base path=w419, name or relative path="data\\sys.ini" ("名称或相对路径")) -> (appended path=w417:path)
            n259 = call <vilib>:"Open Config Data.vi"("configuration file path"=w417) -> ("error out"=w413:errorcluster, "refnum"=w416:T11)  [unwired: 8 in, 1 out]
            n260 = vi-ref "多参数断电保存全局变量.vi"() -> (w415:refnum<vi>)
            n261 = call <userlib>:"Write Panel to INI__ogtk.vi"("error in (no error)"=w413, "VI ref"=w415, "refnum"=w416) -> ("error out"=w412:errorcluster, "refnum out"=w414:T11)  [unwired: 7 in]
            n262 = call <vilib>:"Close Config Data.vi"("error in (no error)"=w412, "refnum"=w414) -> ("error out"=w407:errorcluster, "file path"=w406:path)  [unwired: 8 in]
            n263 = Open/Create/Replace File(file path (use dialog)=w406, error in=w407) -> (refnum out=w410:refnum<file>, error out=w411:errorcluster)  [unwired: 4 in, 1 out]
            n264 = Flush File(refnum=w410, error in=w411) -> (refnum out=w409:refnum<file>, error out=w408:errorcluster)
            n265 = Close File(refnum=w409, error in=w408) -> ()  [unwired: 2 out]
          }
        }
      }
      event "质控参数设置": Value Change {
        n266 = event-data() -> ()  [unwired: 1 in, 6 out]
        n267 = global read "多参数断电保存全局变量.vi" "质控参数设置"() -> (w421:T12)
        n268 = call "多参数质控参数设置.vi"("质控参数设置"=w421) -> ("确定 2"=w420:bool, "质控参数设置 2"=w422:T12)  [unwired: 9 in]
        n269 = case shown="真" w420 {
          tunnel: w422 -> [_ w423]
          frame False {
          }
          frame True {
            n270 = flat-sequence {
              tunnel: w423 -> [w424]
              frame #0 {
                n271 = global write "多参数断电保存全局变量.vi" "质控参数设置"(w424) -> ()
              }
              frame #1 {
                n272 = call <vilib>:"Application Directory.vi"() -> ("Application Directory"=w438:path)
                n273 = Build Path(base path=w438, name or relative path="data\\sys.ini" ("名称或相对路径")) -> (appended path=w436:path)
                n274 = call <vilib>:"Open Config Data.vi"("configuration file path"=w436) -> ("error out"=w432:errorcluster, "refnum"=w435:T11)  [unwired: 8 in, 1 out]
                n275 = vi-ref "多参数断电保存全局变量.vi"() -> (w434:refnum<vi>)
                n276 = call <userlib>:"Write Panel to INI__ogtk.vi"("error in (no error)"=w432, "VI ref"=w434, "refnum"=w435) -> ("error out"=w431:errorcluster, "refnum out"=w433:T11)  [unwired: 7 in]
                n277 = call <vilib>:"Close Config Data.vi"("error in (no error)"=w431, "refnum"=w433) -> ("error out"=w426:errorcluster, "file path"=w425:path)  [unwired: 8 in]
                n278 = Open/Create/Replace File(file path (use dialog)=w425, error in=w426) -> (refnum out=w429:refnum<file>, error out=w430:errorcluster)  [unwired: 4 in, 1 out]
                n279 = Flush File(refnum=w429, error in=w430) -> (refnum out=w428:refnum<file>, error out=w427:errorcluster)
                n280 = Close File(refnum=w428, error in=w427) -> ()  [unwired: 2 out]
              }
            }
          }
        }
      }
      event "释放串口": Value Change {
        n281 = event-data() -> ("NewVal"=w439:bool)  [unwired: 1 in, 5 out]
        n282 = case shown="真" w439 {
          frame False {
          }
          frame True {
            n283 = call "多参数通讯.vi"("STEP"=enum16{"open", "read", "write", "close"}."close") -> ("error out"=w440:errorcluster)  [unwired: 8 in, 2 out]
            n284 = case shown="无错误" w440 {
              frame No Error {
                n285 = property on="打开串口" class="Bool (严格)"("DisabledEnum"=T8."Enabled" ("禁用")) -> ()  [unwired: 2 in, 2 out]
              }
              frame Error {
              }
            }
          }
        }
      }
      event "打开串口": Value Change {
        n286 = event-data() -> ("NewVal"=w443:bool)  [unwired: 1 in, 5 out]
        n287 = case shown="真" w443 {
          frame False {
          }
          frame True {
            n288 = call "多参数通讯.vi"("STEP"=enum16{"open", "read", "write", "close"}."open") -> ("error out"=w444:errorcluster)  [unwired: 8 in, 2 out]
            n289 = case shown="错误" w444 {
              tunnel: [T8."Disabled and Grayed Out" ("禁用") T8."Enabled" ("禁用")] -> w446
              frame No Error {
              }
              frame Error {
                n290 = One Button Dialog(message="多参数串口打开失败" ("消息")) -> ()  [unwired: 1 in, 1 out]
              }
            }
            n291 = property on="打开串口" class="Bool (严格)"("DisabledEnum"=w446, "Value"=FALSE ("打开串口")) -> ()  [unwired: 2 in, 2 out]
          }
        }
      }
      event "水样测试": Value Change {
        n292 = event-data() -> ()  [unwired: 1 in, 6 out]
        n293 = global read "多参数断电保存全局变量.vi" "运行周期"() -> (w454:T13)
        n294 = Unbundle By Name(w454) -> ("运行模式"=w453:enum16{"维护模式", "常规模式", "应急模式", "质控模式"})
        n295 = case shown="\"常规模式\", 默认" w453 {
          tunnel: ["M" ("数据类型") "hd" ("数据类型")] -> w451
          frame "维护模式" {
          }
          frame "常规模式", Default {
          }
        }
        n296 = Bundle By Name(cluster=T9 {"测量模式"="水样测试", "数据类型"="N"} ("启动参数"), "数据类型"=w451) -> (w452:T9)
        n297 = Enqueue Element(queue=w456, element=w452) -> ()  [unwired: 2 in, 3 out]
      }
      event "标样核查": Value Change {
        n298 = event-data() -> ()  [unwired: 1 in, 6 out]
        n299 = call "多参数标样核查对话框.vi"() -> ("确认"=w461:bool, "输出参数"=w459:T14)  [unwired: 10 in]
        n300 = case shown="真" w461 {
          tunnel: w460 -> [_ w464]
          tunnel: w459 -> [_ w463]
          frame False {
          }
          frame True {
            n301 = property class="VI"(reference=w464) -> ("Name"=w468:string, "Exec.State"=w466:T15)  [unwired: 1 in, 2 out]
            n302 = Open VI Reference(type specifier VI Refnum (for type only)=refnum<vi> refnum, vi path=w468, options=128 ("选项")) -> (vi reference=w467:refnum<vi>)  [unwired: 3 in, 1 out]
            n303 = case shown="\"Idle\"" w466 {
              tunnel: w467 -> [w471 w479]
              tunnel: [w471 w478] -> w465
              tunnel: w463 -> [_ w476]
              frame "Bad", Default {
                n304 = One Button Dialog(message="仪器已经启动，无需重复启动" ("消息")) -> ()  [unwired: 1 in, 1 out]
              }
              frame "Idle" {
                n305 = global read "多参数断电保存全局变量.vi" "运行周期"() -> (w475:T13)
                n306 = Unbundle By Name(w475) -> ("运行模式"=w474:enum16{"维护模式", "常规模式", "应急模式", "质控模式"})
                n307 = case shown="\"常规模式\", 默认" w474 {
                  tunnel: ["M" ("数据标记表") "N" ("数据标记表")] -> w477
                  frame "维护模式" {
                  }
                  frame "常规模式", Default {
                  }
                }
                n308 = Bundle By Name(cluster=T10 {"测量模式"="标样核查", "数据类型"="N", "输出参数"={"水温"=FALSE, "pH"=FALSE, "DO"=FALSE, "浊度"=FALSE, "电导率"=FALSE, "叶绿素a"=FALSE, "蓝绿藻"=FALSE, "藻密度"=FALSE, "ORP"=FALSE}} ("启动参数"), "数据类型"=w477, "输出参数"=w476) -> (w472:T10)
                n309 = call-by-ref "开始异步调用"(reference=w479, "启动参数"=w472) -> (reference out=w478:refnum<vi>)  [unwired: 12 in, 1 out]
              }
            }
            n310 = Close Reference(reference=w465) -> ()  [unwired: 1 in, 1 out]
          }
        }
      }
      event "停止": Value Change {
        n311 = event-data() -> ()  [unwired: 1 in, 6 out]
        n312 = Two Button Dialog(message="请再一次确认是否停止测量" ("消息")) -> (T button?=w482:bool)  [unwired: 2 in]
        n313 = case shown="真" w482 {
          tunnel: w484 -> [_ w487]
          frame False {
          }
          frame True {
            w485 = u16 11 items=["启动测量（全部）"=1, "初始化（清洗）"=10, "停止测量（全部）"=11, "校时"=13, "启动测量（单个传感器）"=19, "停止测量（单个传感器）"=20] ("控制命令")
            w486 = u16 10 items=["氨氮"=3, "水温"=9, "pH值"=10, "溶解氧"=11, "电导率"=12, "浊度"=13, "叶绿素a"=14, "藻密度"=15, "蓝绿藻"=16, "氧化还原电位"=17, "溶解氧%"=18, "盐度"=19] ("站号")
            n314 = Send Notification(notification=TRUE ("通知"), notifier=w487) -> ()  [unwired: 1 in, 2 out]
            n315 = call "多参数控制命令.vi"("控制命令"=w485, "站号"=w486) -> ()  [unwired: 9 in, 1 out]
          }
        }
      }
      event "设置": Value Change {
        n316 = event-data() -> ()  [unwired: 1 in, 6 out]
        n317 = property on="窗格" class="Pane"("Origin"=T2 {"Horizontal"=0, "Vertical"=628} ("原点")) -> ()  [unwired: 2 in, 2 out]
      }
      event "返回": Value Change {
        n318 = event-data() -> ()  [unwired: 1 in, 6 out]
        n319 = property on="窗格" class="Pane"("Origin"=T2 {"Horizontal"=0, "Vertical"=0} ("原点")) -> ()  [unwired: 2 in, 2 out]
      }
      event "传感器参数读取", "获取传感器参数并保存触发": Value Change {
        n320 = event-data() -> ()  [unwired: 1 in, 6 out]
        n321 = call "多参数传感器参数读取.vi"() -> ("error out"=w494:errorcluster, "modbus"=w492:u16[], "添加的数组"=w493:string[][])  [unwired: 9 in]
        n322 = property on="传感器区" class="MCListbox (严格)"("ItemNames"=w493) -> ()  [unwired: 2 in, 2 out]
        n323 = call <vilib>:"General Error Handler.vi"("error in (no error)"=w494) -> ("error out"=w491:errorcluster)  [unwired: 10 in, 4 out]
        n324 = case shown="无错误" w491 {
          tunnel: w492 -> [w495 _]
          frame No Error {
            n325 = flat-sequence {
              tunnel: w495 -> [w496]
              frame #0 {
                n326 = global write "多参数断电保存全局变量.vi" "传感器参数modbus"(w496) -> ()
              }
              frame #1 {
                n327 = call "配置保存.vi"() -> ()  [unwired: 11 in, 1 out]
              }
            }
          }
          frame Error {
          }
        }
      }
      event "关键参数区读取": Value Change {
        n328 = event-data() -> ()  [unwired: 1 in, 6 out]
        n329 = call "多参数关键参数读取.vi"() -> ("error out"=w497:errorcluster, "添加的数组"=w498:string[][])  [unwired: 10 in]
        n330 = call <vilib>:"General Error Handler.vi"("error in (no error)"=w497) -> ()  [unwired: 10 in, 5 out]
        n331 = property on="关键参数区" class="MCListbox (严格)"("ItemNames"=w498) -> ()  [unwired: 2 in, 2 out]
      }
      event "同步时间": Value Change {
        w499 = u16 13 items=["启动测量（全部）"=1, "初始化（清洗）"=10, "停止测量（全部）"=11, "校时"=13, "启动测量（单个传感器）"=19, "停止测量（单个传感器）"=20] ("控制命令")
        w500 = u16 9 items=["氨氮"=3, "水温"=9, "pH值"=10, "溶解氧"=11, "电导率"=12, "浊度"=13, "叶绿素a"=14, "藻密度"=15, "蓝绿藻"=16, "氧化还原电位"=17, "溶解氧%"=18, "盐度"=19] ("站号")
        n332 = event-data() -> ()  [unwired: 1 in, 6 out]
        n333 = call "多参数控制命令.vi"("控制命令"=w499, "站号"=w500) -> ("error out"=w502:errorcluster)  [unwired: 9 in]
        n334 = case shown="错误" w502 {
          tunnel: ["时间同步成功" ("消息") "时间同步失败" ("消息")] -> w501
          frame No Error {
          }
          frame Error {
          }
        }
        n335 = One Button Dialog(message=w501) -> ()  [unwired: 1 in, 1 out]
      }
      event "启动测量(全部)": Value Change {
        w505 = u16 1 items=["启动测量（全部）"=1, "初始化（清洗）"=10, "停止测量（全部）"=11, "校时"=13, "启动测量（单个传感器）"=19, "停止测量（单个传感器）"=20] ("控制命令")
        w506 = u16 9 items=["氨氮"=3, "水温"=9, "pH值"=10, "溶解氧"=11, "电导率"=12, "浊度"=13, "叶绿素a"=14, "藻密度"=15, "蓝绿藻"=16, "氧化还原电位"=17, "溶解氧%"=18, "盐度"=19] ("站号")
        n336 = event-data() -> ()  [unwired: 1 in, 6 out]
        n337 = call "多参数控制命令.vi"("控制命令"=w505, "站号"=w506) -> ("error out"=w508:errorcluster)  [unwired: 9 in]
        n338 = case shown="无错误" w508 {
          tunnel: ["启动成功" ("消息") "启动失败" ("消息")] -> w507
          frame No Error {
          }
          frame Error {
          }
        }
        n339 = One Button Dialog(message=w507) -> ()  [unwired: 1 in, 1 out]
      }
      event "停止测量(全部)": Value Change {
        w513 = u16 11 items=["启动测量（全部）"=1, "初始化（清洗）"=10, "停止测量（全部）"=11, "校时"=13, "启动测量（单个传感器）"=19, "停止测量（单个传感器）"=20] ("控制命令")
        w514 = u16 9 items=["氨氮"=3, "水温"=9, "pH值"=10, "溶解氧"=11, "电导率"=12, "浊度"=13, "叶绿素a"=14, "藻密度"=15, "蓝绿藻"=16, "氧化还原电位"=17, "溶解氧%"=18, "盐度"=19] ("站号")
        n340 = event-data() -> ()  [unwired: 1 in, 6 out]
        n341 = call "多参数控制命令.vi"("控制命令"=w513, "站号"=w514) -> ("error out"=w512:errorcluster)  [unwired: 9 in]
        n342 = case shown="错误" w512 {
          tunnel: ["停止成功" ("消息") "停止失败" ("消息")] -> w511
          frame No Error {
          }
          frame Error {
          }
        }
        n343 = One Button Dialog(message=w511) -> ()  [unwired: 1 in, 1 out]
      }
      event "初始化(清洗)": Value Change {
        w519 = u16 10 items=["启动测量（全部）"=1, "初始化（清洗）"=10, "停止测量（全部）"=11, "校时"=13, "启动测量（单个传感器）"=19, "停止测量（单个传感器）"=20] ("控制命令")
        w520 = u16 9 items=["氨氮"=3, "水温"=9, "pH值"=10, "溶解氧"=11, "电导率"=12, "浊度"=13, "叶绿素a"=14, "藻密度"=15, "蓝绿藻"=16, "氧化还原电位"=17, "溶解氧%"=18, "盐度"=19] ("站号")
        n344 = event-data() -> ()  [unwired: 1 in, 6 out]
        n345 = call "多参数控制命令.vi"("控制命令"=w519, "站号"=w520) -> ("error out"=w517:errorcluster)  [unwired: 9 in]
        n346 = case shown="错误" w517 {
          tunnel: ["初始化成功" ("消息") "初始化失败" ("消息")] -> w518
          frame No Error {
          }
          frame Error {
          }
        }
        n347 = One Button Dialog(message=w518) -> ()  [unwired: 1 in, 1 out]
      }
      event "启动测量(单探)": Value Change {
        w523 = u16 19 items=["启动测量（全部）"=1, "初始化（清洗）"=10, "停止测量（全部）"=11, "校时"=13, "启动测量（单个传感器）"=19, "停止测量（单个传感器）"=20] ("控制命令")
        n348 = event-data() -> ()  [unwired: 1 in, 6 out]
        n349 = property class="Ring (严格)"(reference=w527) -> ("Value"=w526:u16)  [unwired: 1 in, 2 out]
        n350 = call "多参数控制命令.vi"("控制命令"=w523, "站号"=w526) -> ("error out"=w525:errorcluster)  [unwired: 9 in]
        n351 = case shown="无错误" w525 {
          tunnel: ["启动成功" ("消息") "启动失败" ("消息")] -> w524
          frame No Error {
          }
          frame Error {
          }
        }
        n352 = One Button Dialog(message=w524) -> ()  [unwired: 1 in, 1 out]
      }
      event "停止测量(单探)": Value Change {
        w530 = u16 20 items=["启动测量（全部）"=1, "初始化（清洗）"=10, "停止测量（全部）"=11, "校时"=13, "启动测量（单个传感器）"=19, "停止测量（单个传感器）"=20] ("控制命令")
        n353 = event-data() -> ()  [unwired: 1 in, 6 out]
        n354 = property class="Ring (严格)"(reference=w534) -> ("Value"=w533:u16)  [unwired: 1 in, 2 out]
        n355 = call "多参数控制命令.vi"("控制命令"=w530, "站号"=w533) -> ("error out"=w532:errorcluster)  [unwired: 9 in]
        n356 = case shown="错误" w532 {
          tunnel: ["停止成功" ("消息") "停止失败" ("消息")] -> w531
          frame No Error {
          }
          frame Error {
          }
        }
        n357 = One Button Dialog(message=w531) -> ()  [unwired: 1 in, 1 out]
      }
    }
  }
